vi "Send Increment.vi"(7 "Message Priority":T1=enum."Normal", 8 "error in (no error)":errorcluster, 10 "Numeric":dbl, 11 "Actor Framework.lvlib:Send Queue":refnum<class "Message Enqueuer.lvclass">) -> (0 "error out":errorcluster)   [LabVIEW 2020, in "Messaging Tests.lvlib" / "Increment Msg.lvclass"]
uses:
  Increment Msg.lvclass
  vi.lib/ActorFramework/Message Enqueuer/Message Enqueuer.lvclass
  C:/dev/actor-framework/dist/vi.lib/ActorFramework/Message/Message.lvclass
  Increment Msg.lvclass/Increment Msg.ctl
  vi.lib/ActorFramework/Message Enqueuer/Message Enqueuer.lvclass/Message Enqueuer.ctl
  vi.lib/ActorFramework/Message Enqueuer/Message Priority.ctl
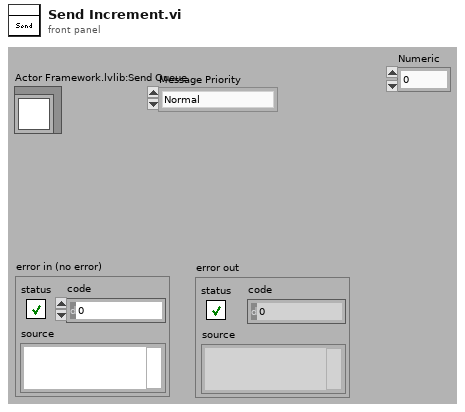
[diagram p1: front panel]
types:
  T1 = typedef "Actor Framework.lvlib/Message Enqueuer.lvclass/Message Priority.ctl" = enum16{"Low", "Normal", "High"}
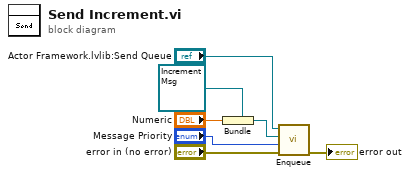
[diagram p0: block diagram]
diagram:
  n1 = Bundle(cluster=refnum<class "Increment Msg.lvclass"> refnum ("Object"), "Numeric") -> (w3:refnum<class "Increment Msg.lvclass">)
  n2 = call "Enqueue.vi"("error in (no error)"="error in (no error)", "Message Priority (Normal)"="Message Priority", "Message"=w3, "Message Enqueuer in"="Actor Framework.lvlib:Send Queue") -> ("error out"=→"error out":errorcluster)  [unwired: 6 in, 1 out]
